vi "LVFunction_Imop_CameraSetupFile_GetInformation.vi"(0 "module path":path, 11 "error in (no error)":errorcluster) -> (6 "Camera Config":T1, 15 "error out":errorcluster)   [LabVIEW 2020]
uses:
  CameraSpecifications.ctl
  General dimensions definition.ctl
  Point2D.ctl
  Point2Df.ctl
  Data alignment enum.ctl
  CameraSet.lvclass
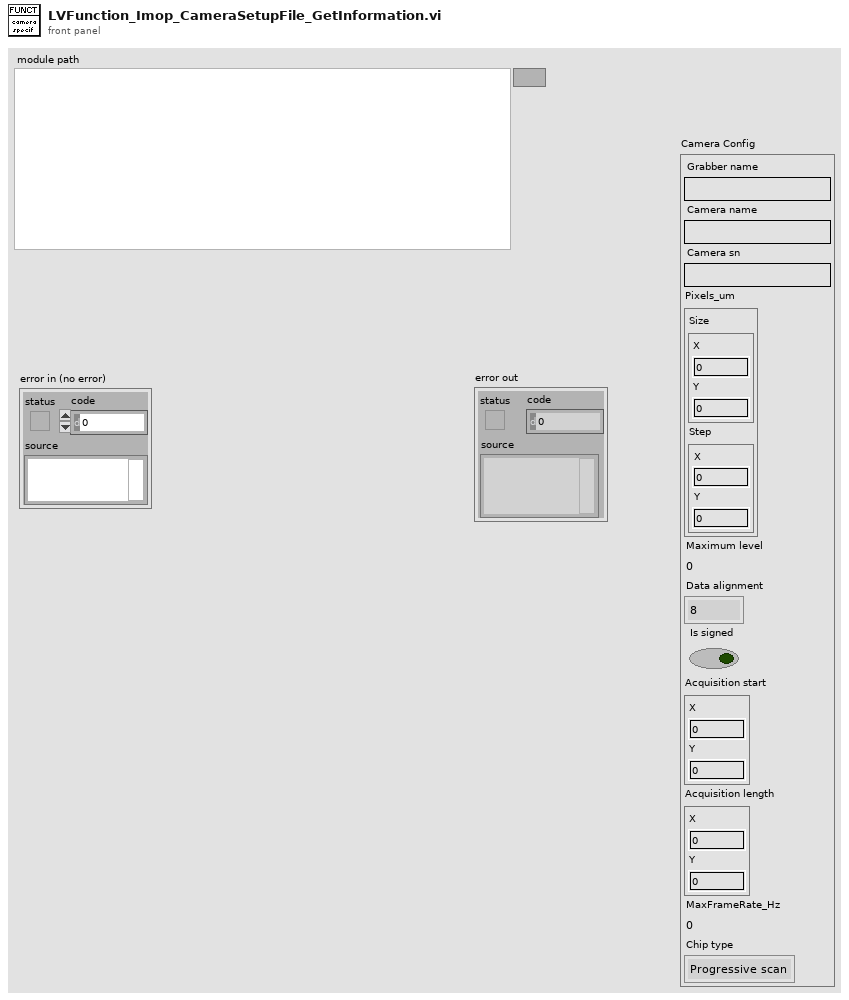
[diagram p1: front panel]
types:
  T1 = typedef "CameraSpecifications.ctl" = cluster{"Grabber name":string, "Camera name":string, "Camera sn":string, "Pixels_um":T2, "Maximum level":u32, "Data alignment":T5, "Is signed":bool, "Acquisition start":T3, "Acquisition length":T3, "MaxFrameRate_Hz":sgl, "Chip type":enum16{"Progressive scan", "Frame transfert"}}
  T2 = typedef "General dimensions definition.ctl" = cluster{"Size":T3, "Step":T4}
  T3 = typedef "Point2D.ctl" = cluster{"X":u32, "Y":u32}
  T4 = typedef "Point2Df.ctl" = cluster{"X":sgl, "Y":sgl}
  T5 = typedef "Data alignment enum.ctl" = enum16{"8", "16", "32"}
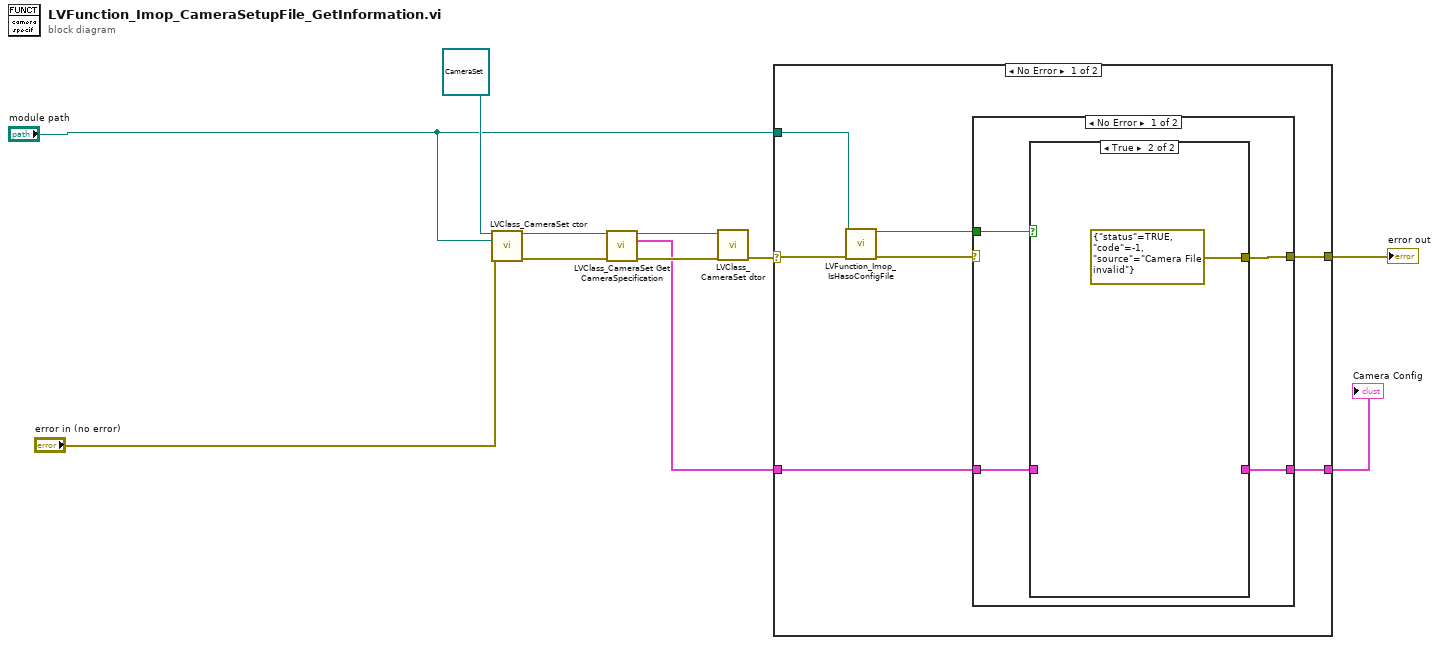
[diagram p0: block diagram]
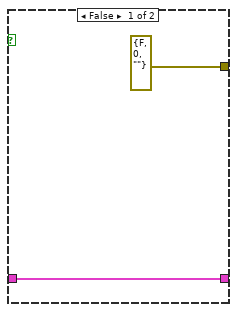
[diagram p2: hidden frame]
diagram:
  n1 = call "LVClass_CameraSet ctor.vi"("CameraSet (const)"=refnum<class "CameraSet.lvclass"> refnum ("CameraSet.lvclass"), "Configuration file path"="module path", "error in (no error)"="error in (no error)") -> ("CameraSet (new)"=w10:refnum<class "CameraSet.lvclass">, "error out"=w9:errorcluster)  [unwired: 11 in]
  n2 = call "LVClass_CameraSet Get CameraSpecification.vi"("CameraSet in"=w10, "error in (no error)"=w9) -> ("CameraSet out"=w8:refnum<class "CameraSet.lvclass">, "Camera Config"=w2:T1, "error out"=w7:errorcluster)  [unwired: 11 in]
  n3 = call "LVClass_CameraSet dtor.vi"("CameraSet in"=w8, "error in (no error)"=w7) -> ("error out"=w6:errorcluster)  [unwired: 12 in, 1 out]
  n4 = case shown="No Error" w6 {
    selector: w6 -> [w13 w27]
    tunnel: [w18 w27] -> w5
    tunnel: w2 -> [w17 _]
    tunnel: [w16 _] -> w4
    tunnel: "module path" -> [w15 _]
    frame No Error {
      n5 = call "LVFunction_Imop_IsHasoConfigFile.vi"("Configuration file path"=w15, "error in"=w13) -> ("IsHasoConfigFile"=w14:bool, "error out"=w12:errorcluster)  [unwired: 12 in]
      n6 = case shown="No Error" w12 {
        selector: w12 -> [_ w26]
        tunnel: [w22 w26] -> w18
        tunnel: w17 -> [w21 _]
        tunnel: [w20 _] -> w16
        tunnel: w14 -> [w19 _]
        frame No Error {
          n7 = case shown="True" w19 {
            tunnel: [errorcluster {"status"=FALSE, "code"=0, "source"=""} ("error out") errorcluster {"status"=TRUE, "code"=-1, "source"="Camera File invalid"} ("error out")] -> w22
            tunnel: [w23 _] -> w20
            tunnel: w21 -> [w23 _]
            frame False {
            }
            frame True {
            }
          }
        }
        frame Error {
        }
      }
    }
    frame Error {
    }
  }
  "error out" <- w5
  "Camera Config" <- w4
